vi "Picture_Exposure_Time.vi"(6 "Pulse per Wavelength":u8[](array[numeric]), 7 "Exposure Time":u32[][](array[numeric]), 8 "Blanking Out":tag="Dev2/port0", 9 "Picture Clock Main in":tag="/Dev1/PFI1", 10 "Number of Pulses per Picture / [x1 us]":i32, 11 "Number of active Koheras lines":i8) -> (0 "error out":errorcluster, 3 "task out":refnum<k21>)   [LabVIEW 2009]
uses:
  <vilib>/DAQmx/write.llb/DAQmx Write (Digital 1D U32 1Chan NSamp).vi
  <vilib>/DAQmx/configure/timing.llb/DAQmx Timing (Sample Clock).vi
  <vilib>/DAQmx/create/channels.llb/DAQmx Create Channel (DO-Digital Output).vi
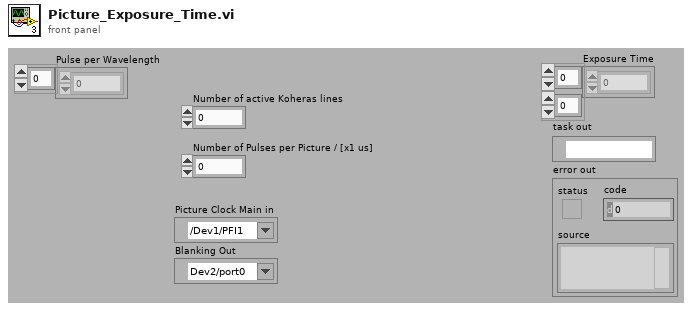
[diagram p1: front panel]
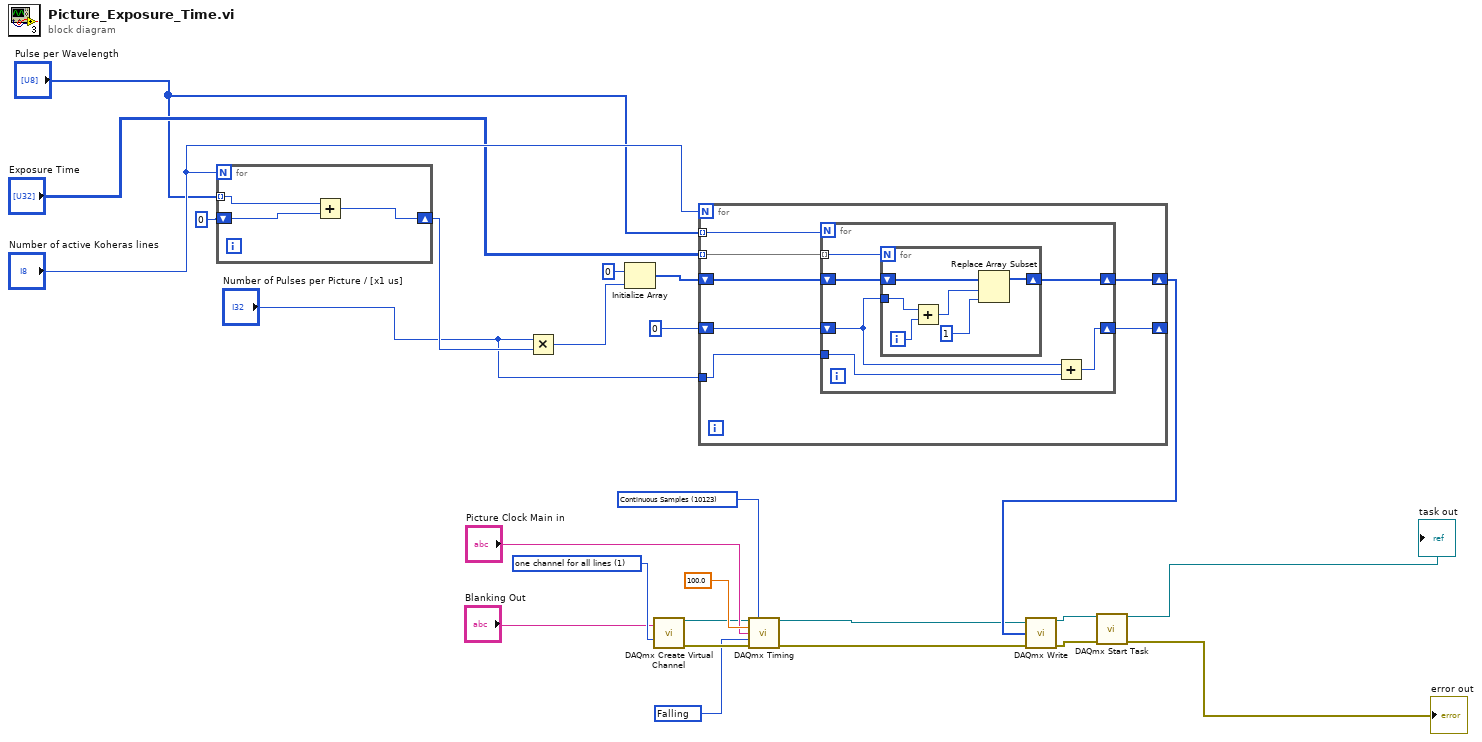
[diagram p0: block diagram]
diagram:
  w16 = 10171 items=["Rising"=10280, "Falling"=10171] ("active edge")
  w25 = 10123 items=["Finite Samples"=10178, "Continuous Samples"=10123, "Hardware Timed Single Point"=12522] ("sample mode")
  w18 = 1 items=["one channel for each line", "one channel for all lines"] ("line grouping")
  n1 = for {
    N: "Number of active Koheras lines" -> [_]
    tunnel: "Pulse per Wavelength" -> [w26] mode=indexing
    shift-right: [w28] -> w10
    shift-left: 0 -> [w27]
    n2 = Add(x=w26, y=w27) -> (x+y=w28:i32)
  }
  n3 = Multiply(x="Number of Pulses per Picture / [x1 us]", y=w10) -> (x*y=w8:i32)
  n4 = Initialize Array(u32 0 ("element"), w8) -> (w12:u32[])
  n5 = call-poly <vilib>:"DAQmx Create Virtual Channel.vi"("lines"="Blanking Out", "line grouping"=w18) -> ("task out"=w19:refnum<k21>, "error out"=w20:errorcluster)  [unwired: 5 in, 7 out]
  n6 = for {
    N: "Number of active Koheras lines" -> [_]
    shift-right: [w34] -> w9
    shift-left: w12 -> [w35]
    tunnel: "Exposure Time" -> [w33] mode=indexing
    tunnel: "Number of Pulses per Picture / [x1 us]" -> [w30]
    shift-right: [w31] -> _
    shift-left: u32 0 ("element") -> [w32]
    tunnel: "Pulse per Wavelength" -> [w29] mode=indexing
    n7 = for {
      N: w29 -> [_]
      shift-right: [w39] -> w34
      shift-left: w35 -> [w40]
      tunnel: w33 -> [w41] mode=indexing
      shift-right: [w38] -> w31
      shift-left: w32 -> [w36]
      tunnel: w30 -> [w37]
      n8 = for {
        N: w41 -> [_]
        shift-right: [w46] -> w39
        shift-left: w40 -> [w47]
        tunnel: w36 -> [w42]
        i -> [w44]
        n9 = Add(x=w42, y=w44) -> (x+y=w43:u32)
        n10 = Replace Array Subset(array=w47, new element=u32 1 ("new element/subarray"), index=w43) -> (w46:u32[])
      }
      n11 = Add(x=w36, y=w37) -> (x+y=w38:u32)
    }
  }
  n12 = call-poly <vilib>:"DAQmx Timing.vi"("task/channels in"=w19, "sample mode"=w25, "rate"=100.0, "source"="Picture Clock Main in", "active edge"=w16, "error in"=w20) -> ("task out"=w1:refnum<k21>, "error out"=w2:errorcluster)  [unwired: 1 in, 7 out]
  n13 = call-poly <vilib>:"DAQmx Write.vi"("task/channels in"=w1, "data"=w9, "error in"=w2) -> ("task out"=w22:refnum<k21>, "error out"=w23:errorcluster)  [unwired: 1 in, 10 out]
  n14 = call <vilib>:"DAQmx Start Task.vi"("task/channels in"=w22, "error in"=w23) -> ("task out"=→"task out":refnum<k21>, "error out"=→"error out":errorcluster)  [unwired: 12 out]
